vi "Execute Command.vi"(8 "error in (no error)":errorcluster, 10 "command":T2={"Command"=enum."Rx", "Parameters"={"arg1"=0, "arg2"=0}}, 11 "Dispatcher in":refnum<class "Dispatcher Thread.lvclass">) -> (0 "error out":errorcluster, 2 "state":T1=enum."Start", 3 "Dispatcher out":refnum<class "Dispatcher Thread.lvclass">)   [LabVIEW 2019, in "DSF Core.lvlib" / "Dispatcher Thread.lvclass"]
uses:
  Dispatcher Thread.lvclass
  Interface/Dispatcher/Command Data.ctl
  Interface/Dispatcher/Command.ctl
  Interface/Dispatcher/Parameters.ctl
  Interface/Dispatcher/Dispatcher Interface.lvclass
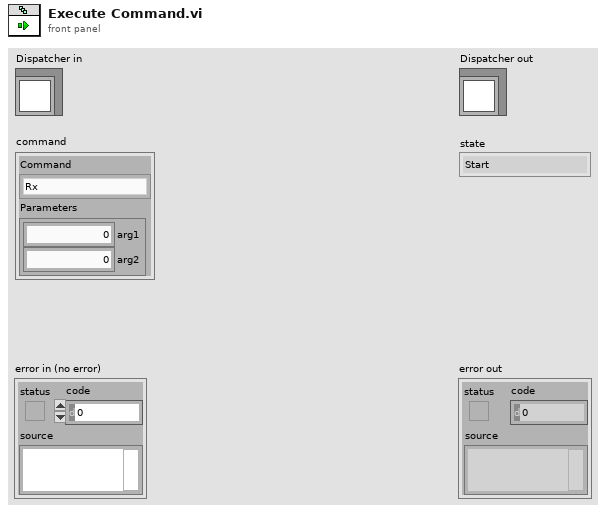
[diagram p1: front panel]
types:
  T1 = typedef "DSF Core.lvlib/Dispatcher Interface.lvclass/Command.ctl" = enum8{"Idle", "Start", "Rx", "Tx", "Set Inline Buffer", "Shutdown", "Error"}
  T2 = typedef "DSF Core.lvlib/Dispatcher Interface.lvclass/Command Data.ctl" = cluster{"Command":T1, "Parameters":T3}
  T3 = typedef "DSF Core.lvlib/Dispatcher Interface.lvclass/Parameters.ctl" = cluster{"arg1":u64, "arg2":u64}
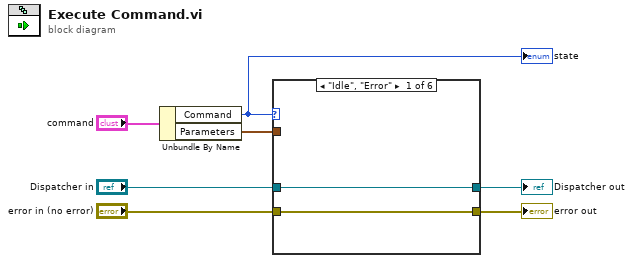
[diagram p0: block diagram]
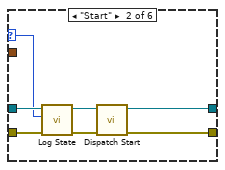
[diagram p2: hidden frame]
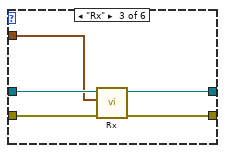
[diagram p3: hidden frame]
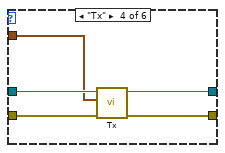
[diagram p4: hidden frame]
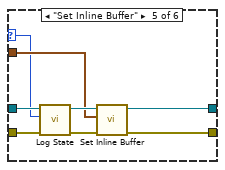
[diagram p5: hidden frame]
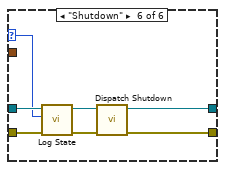
[diagram p6: hidden frame]
diagram:
  n1 = Unbundle By Name("command") -> ("Command"=w1:T1, "Parameters"=w4:T3)
  "state" <- w1
  n2 = case shown="\"Idle\", \"Error\"" w1 {
    selector: w1 -> [_ w10 _ _ w27 w35]
    tunnel: "Dispatcher in" -> [w9 w14 w19 w23 w32 w39]
    tunnel: [w9 w16 w21 w26 w34 w41] -> w3
    tunnel: "error in (no error)" -> [w8 w13 w18 w24 w31 w38]
    tunnel: [w8 w15 w20 w25 w33 w40] -> w2
    tunnel: w4 -> [_ _ w17 w22 w28 _]
    frame "Idle", "Error" {
    }
    frame "Start" {
      n3 = call "Log State.vi"("error in (no error)"=w13, "state"=w10, "Dispatcher in"=w14) -> ("error out"=w11:errorcluster, "Dispatcher out"=w12:refnum<class "Dispatcher Thread.lvclass">)  [unwired: 7 in]
      n4 = call "Dispatch Start.vi"("error in (no error)"=w11, "Dispatcher in"=w12) -> ("error out"=w15:errorcluster, "Dispatcher out"=w16:refnum<class "Dispatcher Thread.lvclass">)  [unwired: 8 in]
    }
    frame "Rx" {
      n5 = call "Rx.vi"("error in (no error)"=w18, "Command Parameters"=w17, "Dispatcher in"=w19) -> ("error out"=w20:errorcluster, "Dispatcher out"=w21:refnum<class "Dispatcher Thread.lvclass">)  [unwired: 7 in]
    }
    frame "Tx" {
      n6 = call "Tx.vi"("error in (no error)"=w24, "Command Parameters"=w22, "Dispatcher in"=w23) -> ("error out"=w25:errorcluster, "Dispatcher out"=w26:refnum<class "Dispatcher Thread.lvclass">)  [unwired: 7 in]
    }
    frame "Set Inline Buffer" {
      n7 = call "Log State.vi"("error in (no error)"=w31, "state"=w27, "Dispatcher in"=w32) -> ("error out"=w29:errorcluster, "Dispatcher out"=w30:refnum<class "Dispatcher Thread.lvclass">)  [unwired: 7 in]
      n8 = call "Set Inline Buffer.vi"("error in (no error)"=w29, "Command Parameters"=w28, "Dispatcher in"=w30) -> ("error out"=w33:errorcluster, "Dispatcher out"=w34:refnum<class "Dispatcher Thread.lvclass">)  [unwired: 7 in]
    }
    frame "Shutdown" {
      n9 = call "Log State.vi"("error in (no error)"=w38, "state"=w35, "Dispatcher in"=w39) -> ("error out"=w36:errorcluster, "Dispatcher out"=w37:refnum<class "Dispatcher Thread.lvclass">)  [unwired: 7 in]
      n10 = call "Dispatch Shutdown.vi"("error in (no error)"=w36, "Dispatcher in"=w37) -> ("error out"=w40:errorcluster, "Dispatcher out"=w41:refnum<class "Dispatcher Thread.lvclass">)  [unwired: 8 in]
    }
  }
  "error out" <- w2
  "Dispatcher out" <- w3
